vi "Send New Message.vi"(7 "Message Priority (Normal)":T1=enum."Normal", 8 "error in (no error)":errorcluster, 9 "New Message":string, 10 "From":string, 11 "Message Enqueuer":refnum<class "Message Enqueuer.lvclass">) -> (0 "error out":errorcluster, 3 "Message Enqueuer out":refnum<class "Message Enqueuer.lvclass">)   [LabVIEW 2015, in "Chat Window Model.lvlib" / "New Message Msg.lvclass"]
doc: "This VI sends the message to an actor."
uses:
  New Message Msg.lvclass
  <vilib>/ActorFramework/Message Enqueuer/Message Enqueuer.lvclass
  <vilib>/ActorFramework/Message Enqueuer/Message Priority.ctl
  New Message Msg.lvclass/New Message Msg.ctl
  <vilib>/ActorFramework/Message Enqueuer/Message Enqueuer.lvclass/Message Enqueuer.ctl
  <vilib>/ActorFramework/Message Priority Queue/Priority Enqueue.vi
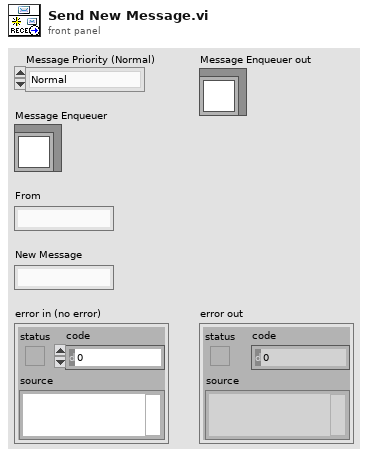
[diagram p1: front panel]
types:
  T1 = typedef "Actor Framework.lvlib/Message Enqueuer.lvclass/Message Priority.ctl" = enum16{"Low", "Normal", "High"}
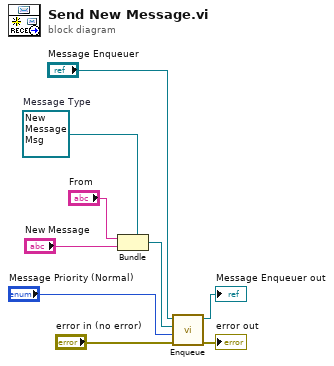
[diagram p0: block diagram]
diagram:
  w3 = refnum<class "New Message Msg.lvclass"> refnum  # Message Type
  n1 = Bundle(cluster=w3, "From", "New Message") -> (w4:refnum<class "New Message Msg.lvclass">)
  n2 = call <vilib>:"Enqueue.vi"("error in (no error)"="error in (no error)", "Message Priority (Normal)"="Message Priority (Normal)", "Message"=w4, "Message Enqueuer in"="Message Enqueuer") -> ("error out"=→"error out":errorcluster, "Message Enqueuer out"=→"Message Enqueuer out":refnum<class "Message Enqueuer.lvclass">)  [unwired: 6 in]
